vi "Poly Set Stepper.vi"   [LabVIEW 2012]
doc: "Sets the stepper motor wired to the specified \"Port\" to the characteristics assigned to \"Variable in\"."
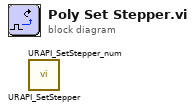
[diagram p0: block diagram]
diagram:
  n1 = call <userlib>:"URAPI_SetStepper.vi"() -> ()  [unwired: 4 in, 2 out]
  n2 = call <userlib>:"URAPI_SetStepper_num.vi"() -> ()  [unwired: 4 in, 2 out]
